vi "CreateNewBoard_RandomSize.vi"(8 "error in (no error)":errorcluster, 9 "MaxBoardSize":u16, 10 "MinBoardSize":u16) -> (0 "error out":errorcluster, 2 "Board out":refnum<class "Board.lvclass">)   [LabVIEW 2015, in "TronviewGame.lvlib" / "GameBuilder.lvclass"]
uses:
  GameBuilder.lvclass
  Board/Board.lvclass
  Board/BoardSize.ctl
  <vilib>/Analysis/1siggen.llb/Ramp Pattern by Delta.vi
  <vilib>/Analysis/1siggen.llb/Riffle Array (DBL).vi
  <vilib>/Analysis/NI_AALBase.lvlib
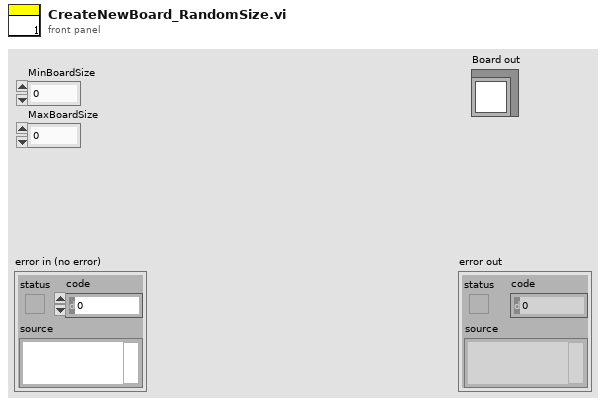
[diagram p1: front panel]
types:
  T1 = typedef "TronviewGame.lvlib/Board.lvclass/BoardSize.ctl" = cluster{"Columns":u16, "Rows":u16}
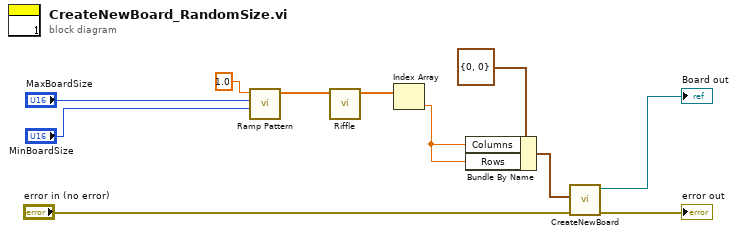
[diagram p0: block diagram]
diagram:
  n1 = call-poly <vilib>:"Ramp Pattern.vi"("start"="MinBoardSize", "end"="MaxBoardSize", "delta"=1.0) -> ("Ramp Pattern"=w6:dbl[])  [unwired: 6 in, 2 out]
  n2 = call-poly <vilib>:"Riffle.vi"("X"=w6) -> ("Riffled {X}"=w5:dbl[])  [unwired: 8 in, 2 out]
  n3 = Index Array(array=w5) -> (element=w4:dbl)  [unwired: 1 in]
  n4 = Bundle By Name(cluster=T1 {"Columns"=0, "Rows"=0} ("Size"), "Columns"=w4, "Rows"=w4) -> (w10:T1)
  n5 = call "CreateNewBoard.vi"("error in (no error)"="error in (no error)", "Size"=w10) -> ("error out"=→"error out":errorcluster, "Board out"=→"Board out":refnum<class "Board.lvclass">)  [unwired: 8 in]
